vi "Timer tengely.vi"(8 "error in (no error)":errorcluster, 11 "Message Queues in":T1) -> (0 "error out":errorcluster, 3 "Message Queue":refnum<queue>)   [LabVIEW 2014]
uses:
  support/Message Queue/Message Queue.lvlib
  support/Message Queue/Enqueue Message (Single).vi
  Engine/Message.ctl
  Teszt/Command.ctl
  Teszt/Teszt.ctl
  <vilib>/ErrorRing/Error Ring.xnode
  <vilib>/Utility/error.llb/Error Cluster From Error Code.vi
  support/Message Queue/Message Cluster.ctl
  support/Message Queue/All Message Queues.ctl
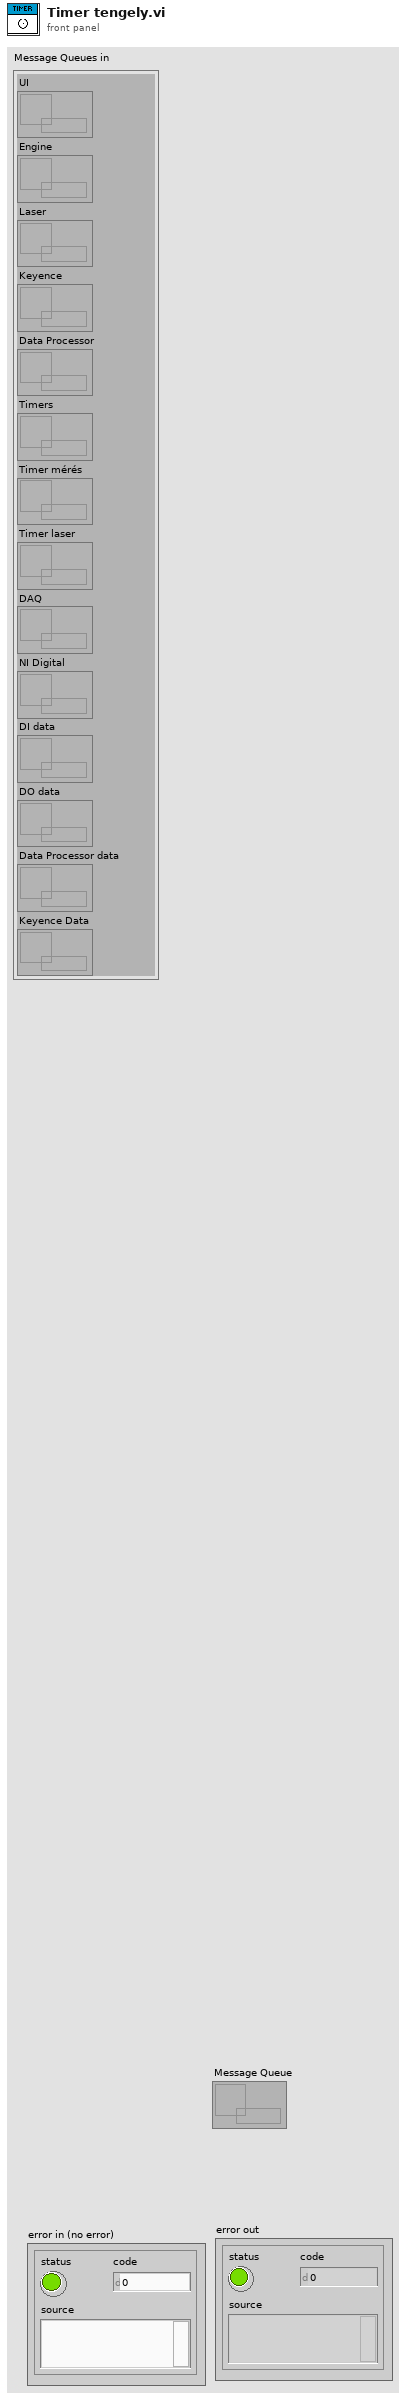
[diagram p1: front panel]
types:
  T1 = typedef "Message Queue.lvlib/All Message Queues.ctl" = cluster{"UI":refnum<queue>, "Engine":refnum<queue>, "Laser":refnum<queue>, "Keyence":refnum<queue>, "Data Processor":refnum<queue>, "Timers":refnum<queue>, "Timer mérés":refnum<queue>, "Timer laser":refnum<queue>, "DAQ":refnum<queue>, "NI Digital":refnum<queue>, "DI data":refnum<queue>, "DO data":refnum<queue>, "Data Processor data":refnum<queue>, "Keyence Data":refnum<queue>}
  T2 = typedef "Teszt.ctl" = cluster{"Thread ID":dbl, "Mérésszám":string, "Mérés/Utasítás":string, "Command":T3, "Min":string, "Max":string, "Aktív?":bool, "Log?":bool, "Kiértékelés":bool, "Etalon 1 exp":bool, "Etalon 2 exp":bool, "Etalon 3 exp":bool, "Etalon 4 exp":bool, "Etalon 5 exp":bool}
  T3 = typedef "Command.ctl" = cluster{"Parancs":string, "Paraméter 1":string, "Paraméter 2":string, "Paraméter 3":string, "Paraméter 4":string, "Paraméter 5":string, "Eredmény":string}
  T4 = typedef "Message.ctl" = cluster{"Thread ID":u16, "Callback":string, "Data":variant, "Error":errorcluster}
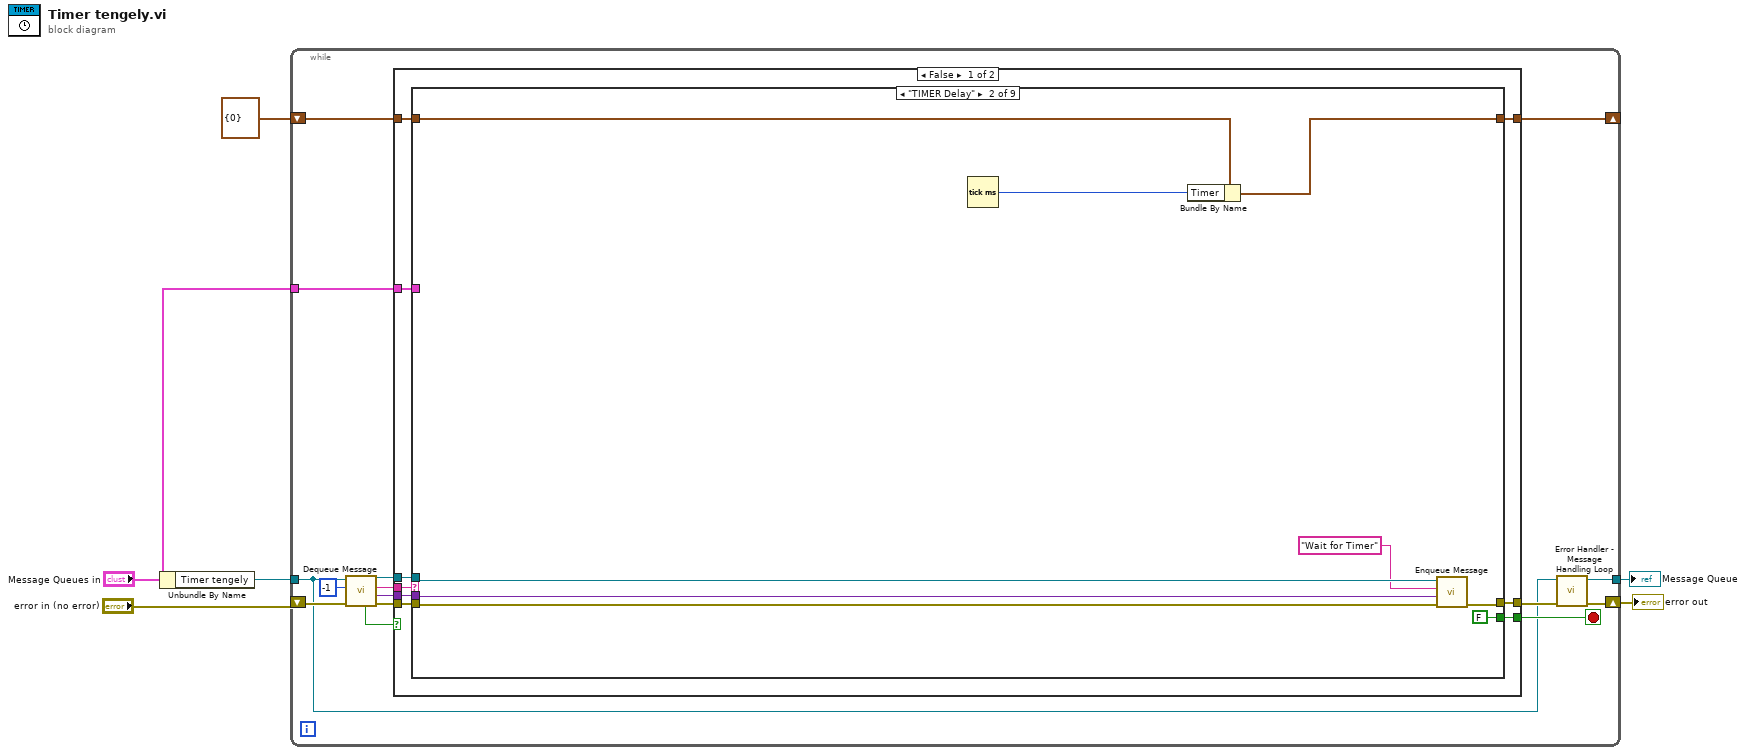
[diagram p0: block diagram]
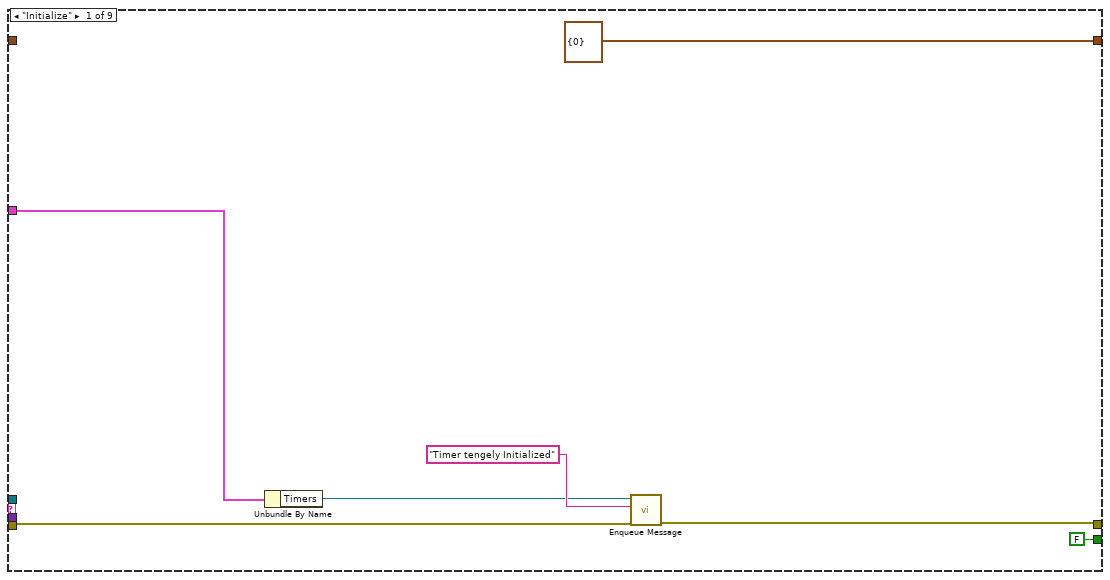
[diagram p2: hidden frame]
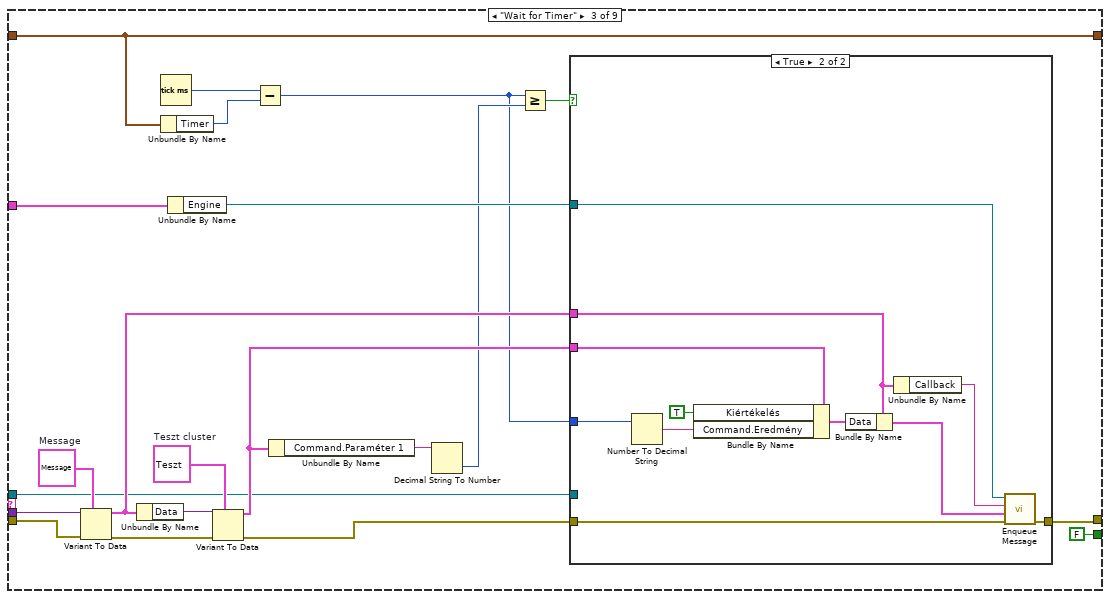
[diagram p3: hidden frame]
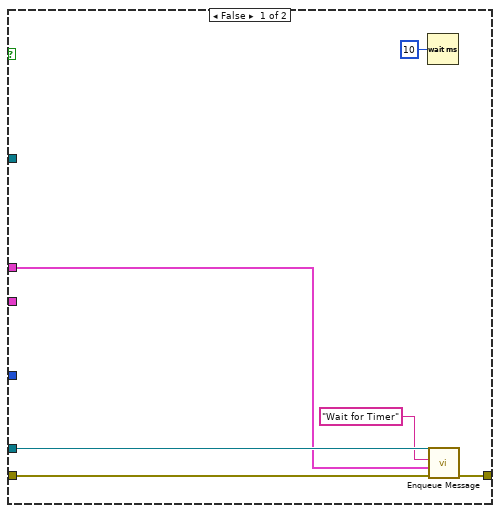
[diagram p4: hidden frame]
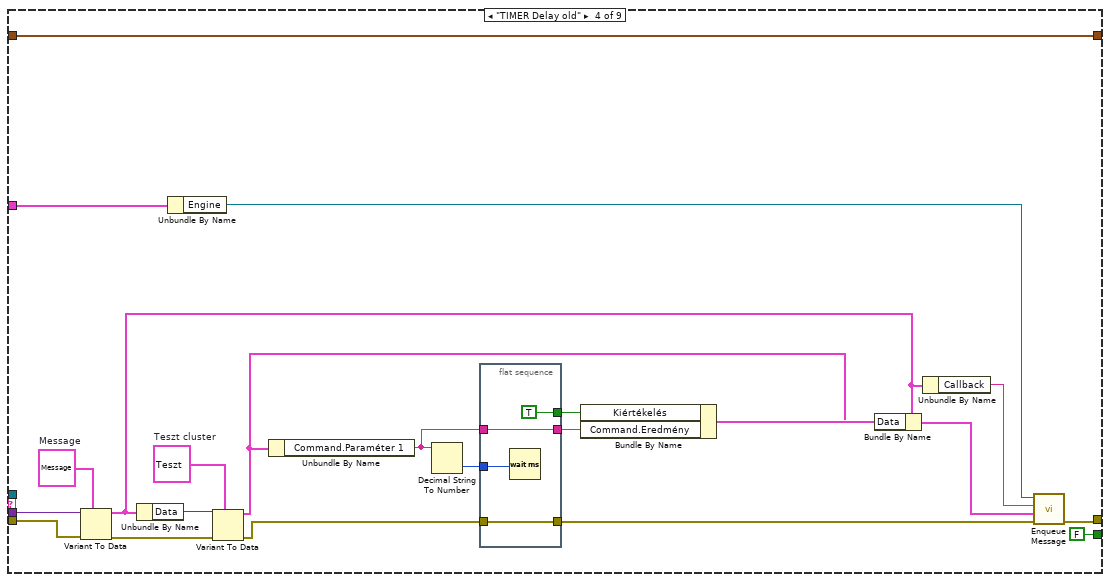
[diagram p5: hidden frame]
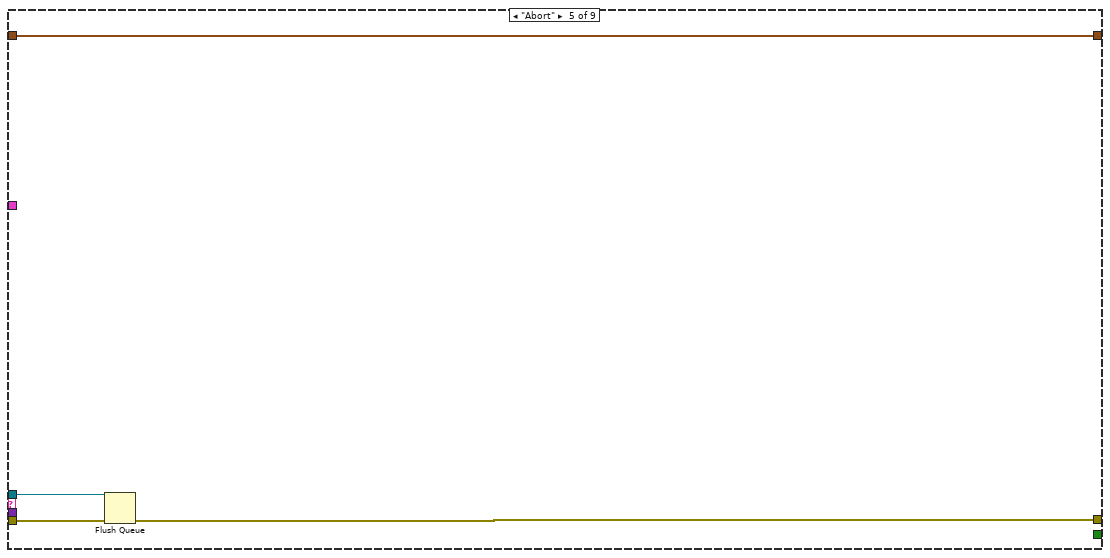
[diagram p6: hidden frame]
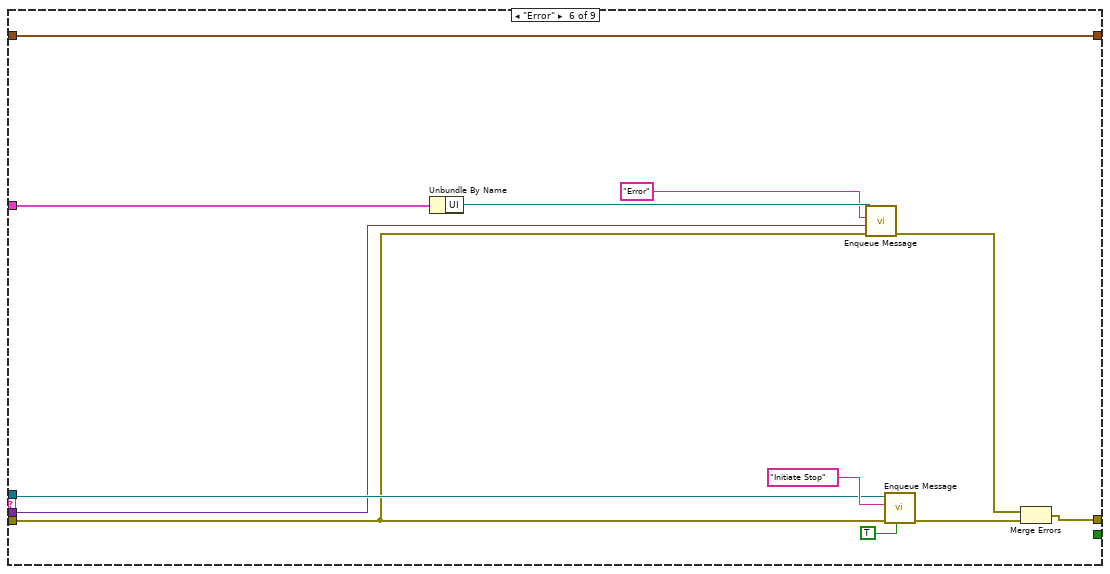
[diagram p7: hidden frame]
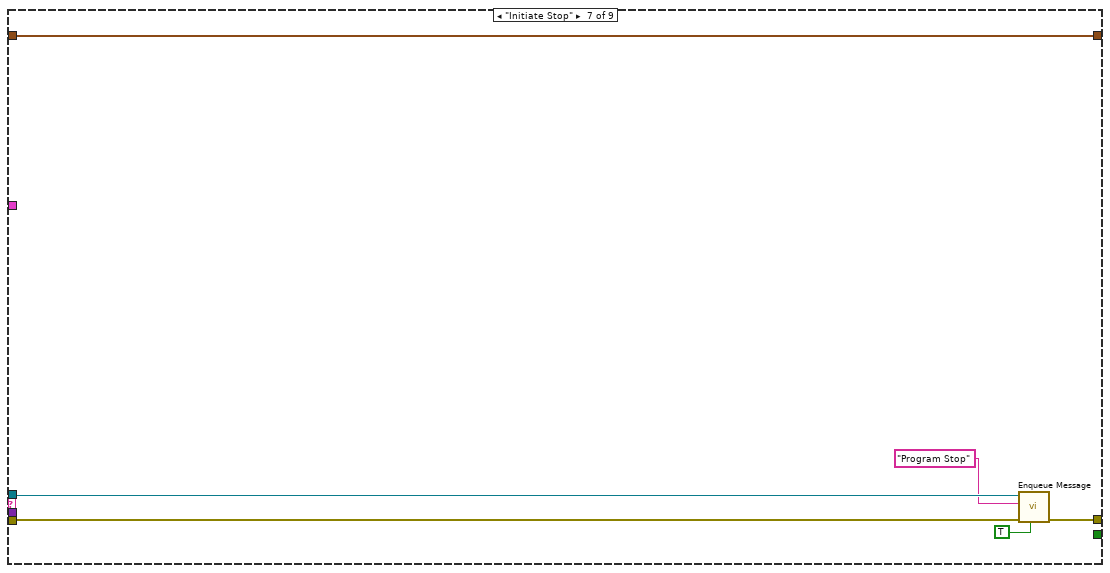
[diagram p8: hidden frame]
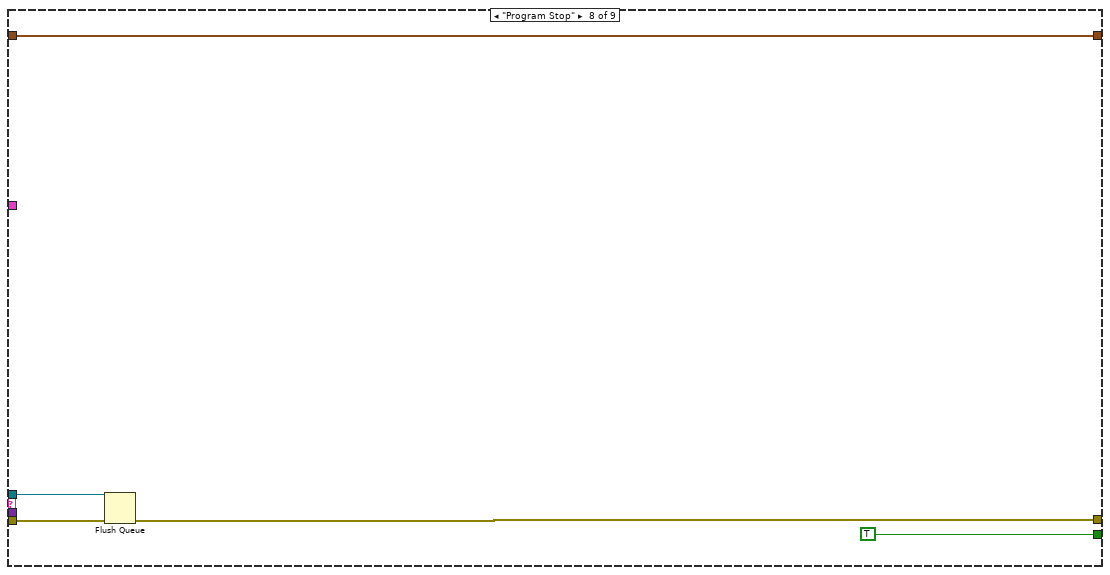
[diagram p9: hidden frame]
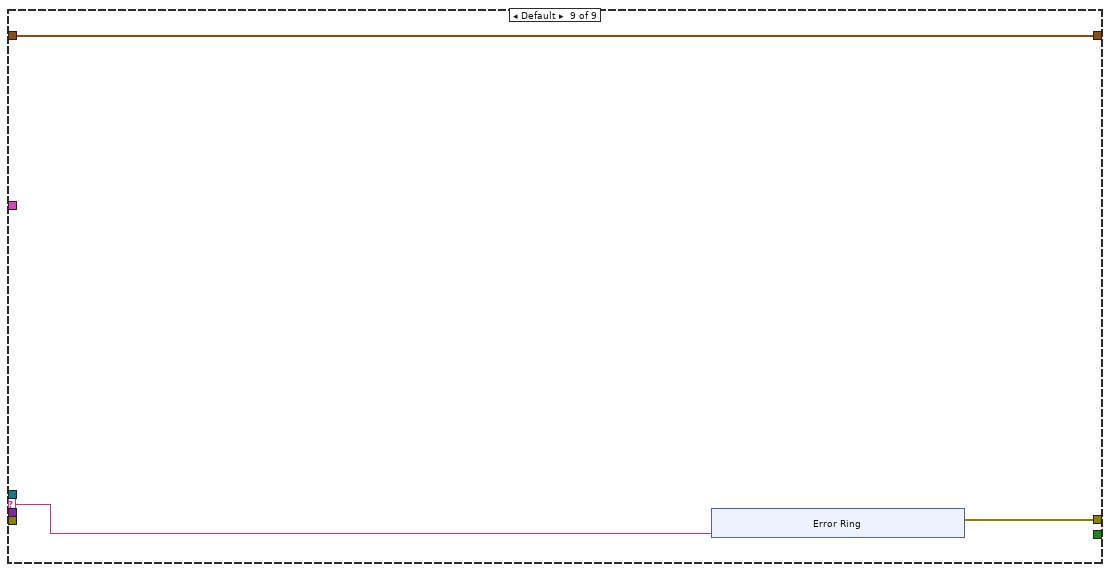
[diagram p10: hidden frame]
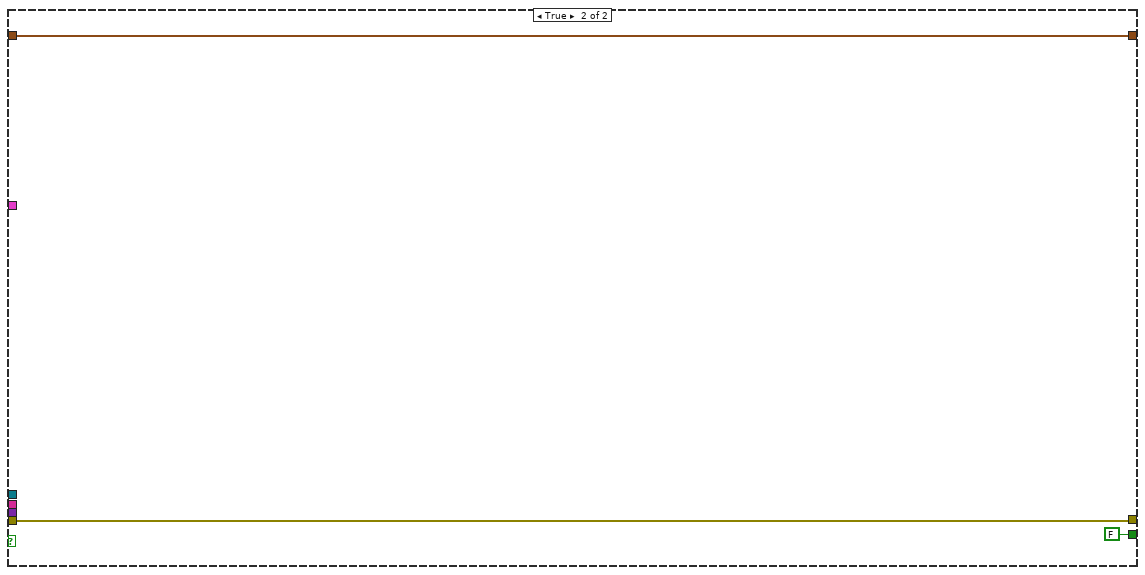
[diagram p11: hidden frame]
diagram:
  n1 = Unbundle By Name("Message Queues in") -> ("Timer tengely"=w3:refnum<queue>)
  n2 = while {
    tunnel: w3 -> [w9]
    shift-right: [w14] -> _
    shift-left: cluster{"Timer":u32} {"Timer"=0} -> [w7]
    shift-right: [w12] -> w6
    shift-left: "error in (no error)" -> [w21]
    tunnel: "Message Queues in" -> [w10]
    tunnel: [w8] -> w2
    stop <- w17 stop-if-true
    n3 = call "Dequeue Message.vi"("error in (no error)"=w21, "timeout in ms (-1)"=-1, "Message Queue"=w9) -> ("error out"=w19:errorcluster, "Message Data"=w13:variant, "Message"=w20:string, "dup Message Queue"=w18:refnum<queue>, "timed out?"=w15:bool)  [unwired: 4 in]
    n4 = case shown="False" w15 {
      tunnel: w20 -> [w30 _]
      tunnel: w19 -> [w29 w149]
      tunnel: w18 -> [w28 _]
      tunnel: [w27 FALSE] -> w17
      tunnel: [w26 w149] -> w11
      tunnel: w7 -> [w24 w150]
      tunnel: [w25 w150] -> w14
      tunnel: w13 -> [w23 _]
      tunnel: w10 -> [w22 _]
      frame False {
        n5 = case shown="\"TIMER Delay\"" w30 {
          selector: w30 -> [_ _ _ _ _ _ _ _ w138]
          tunnel: w29 -> [w33 w42 w67 w106 w114 w116 w130 w137 _]
          tunnel: w28 -> [_ w43 w47 _ w113 w118 w129 w136 _]
          tunnel: [w34 w45 w60 w96 w111 w119 w131 w133 w139] -> w26
          tunnel: [FALSE FALSE FALSE FALSE _ _ _ TRUE _] -> w27
          tunnel: [cluster{"Timer":u32} {"Timer"=0} w38 w54 w105 w112 w126 w132 w134 w140] -> w25
          tunnel: w24 -> [_ w39 w54 w105 w112 w126 w132 w134 w140]
          tunnel: w23 -> [_ w44 w65 w103 _ w115 _ _ _]
          tunnel: w22 -> [w32 _ w57 w92 _ w117 _ _ _]
          frame "Initialize" {
            n6 = Unbundle By Name(w32) -> ("Timers"=w35:refnum<queue>)
            n7 = call-poly "Enqueue Message.vi"("error in (no error)"=w33, "Message"="Timer tengely Initialized", "Message Queue"=w35) -> ("error out"=w34:errorcluster)  [unwired: 7 in, 1 out]
          }
          frame "TIMER Delay" {
            n8 = Tick Count (ms)() -> (millisecond timer value=w40:u32)
            n9 = Bundle By Name(cluster=w39, "Timer"=w40) -> (w38:cluster{"Timer":u32})
            n10 = call-poly "Enqueue Message.vi"("error in (no error)"=w42, "Message Data"=w44, "Message"="Wait for Timer", "Message Queue"=w43) -> ("error out"=w45:errorcluster)  [unwired: 6 in, 1 out]
          }
          frame "Wait for Timer" {
            w61 = T2 {"Thread ID"=0.0, "Mérésszám"="", "Mérés/Utasítás"="", "Command"={"Parancs"="", "Paraméter 1"="", "Paraméter 2"="", "Paraméter 3"="", "Paraméter 4"="", "Paraméter 5"="", "Eredmény"=""}, "Min"="", "Max"="", "Aktív?"=FALSE, "Log?"=FALSE, "Kiértékelés"=FALSE, "Etalon 1 exp"=FALSE, "Etalon 2 exp"=FALSE, "Etalon 3 exp"=FALSE, "Etalon 4 exp"=FALSE, "Etalon 5 exp"=FALSE}  # Teszt cluster
            w64 = T4 {"Thread ID"=0, "Callback"="", "Data"=variant, "Error"={"status"=FALSE, "code"=0, "source"=""}}  # Message
            n11 = Variant To Data(error in=w67, type=w64, Variant=w65) -> (data=w58:T4, error out=w62:errorcluster)
            n12 = Unbundle By Name(w58) -> ("Data"=w63:variant)
            n13 = Tick Count (ms)() -> (millisecond timer value=w53:u32)
            n14 = Unbundle By Name(w54) -> ("Timer"=w52:u32)
            n15 = Unbundle By Name(w57) -> ("Engine"=w56:refnum<queue>)
            n16 = Variant To Data(error in=w62, type=w61, Variant=w63) -> (data=w59:T2, error out=w48:errorcluster)
            n17 = Subtract(x=w53, y=w52) -> (x-y=w50:u32)
            n18 = Unbundle By Name(w59) -> ("Command.Paraméter 1"=w55:string)
            n19 = Decimal String To Number(string=w55) -> (number=w51:i32)  [unwired: 2 in, 1 out]
            n20 = Greater Or Equal?(x=w50, y=w51) -> (x >= y?=w49:bool)
            n21 = case shown="True" w49 {
              tunnel: [w73 w82] -> w60
              tunnel: w59 -> [_ w81]
              tunnel: w58 -> [w69 w80]
              tunnel: w56 -> [_ w78]
              tunnel: w50 -> [_ w74]
              tunnel: w48 -> [w71 w75]
              tunnel: w47 -> [w72 _]
              frame False {
                n22 = Wait (ms)(milliseconds to wait=u32 10) -> ()  [unwired: 1 out]
                n23 = call-poly "Enqueue Message.vi"("error in (no error)"=w71, "Message Data"=w69, "Message"="Wait for Timer", "Message Queue"=w72) -> ("error out"=w73:errorcluster)  [unwired: 6 in, 1 out]
              }
              frame True {
                n24 = Number To Decimal String(number=w74) -> (decimal integer string=w76:string)  [unwired: 1 in]
                n25 = Bundle By Name(cluster=w81, "Kiértékelés"=TRUE, "Command.Eredmény"=w76) -> (w84:T2)
                n26 = Bundle By Name(cluster=w80, "Data"=w84) -> (w83:T4)
                n27 = Unbundle By Name(w80) -> ("Callback"=w79:string)
                n28 = call-poly "Enqueue Message.vi"("error in (no error)"=w75, "Message Data"=w83, "Message"=w79, "Message Queue"=w78) -> ("error out"=w82:errorcluster)  [unwired: 6 in, 1 out]
              }
            }
          }
          frame "TIMER Delay old" {
            w99 = T2 {"Thread ID"=0.0, "Mérésszám"="", "Mérés/Utasítás"="", "Command"={"Parancs"="", "Paraméter 1"="", "Paraméter 2"="", "Paraméter 3"="", "Paraméter 4"="", "Paraméter 5"="", "Eredmény"=""}, "Min"="", "Max"="", "Aktív?"=FALSE, "Log?"=FALSE, "Kiértékelés"=FALSE, "Etalon 1 exp"=FALSE, "Etalon 2 exp"=FALSE, "Etalon 3 exp"=FALSE, "Etalon 4 exp"=FALSE, "Etalon 5 exp"=FALSE}  # Teszt cluster
            w102 = T4 {"Thread ID"=0, "Callback"="", "Data"=variant, "Error"={"status"=FALSE, "code"=0, "source"=""}}  # Message
            n29 = Variant To Data(error in=w106, type=w102, Variant=w103) -> (data=w94:T4, error out=w100:errorcluster)
            n30 = Unbundle By Name(w94) -> ("Data"=w101:variant)
            n31 = Unbundle By Name(w92) -> ("Engine"=w91:refnum<queue>)
            n32 = Variant To Data(error in=w100, type=w99, Variant=w101) -> (data=w95:T2, error out=w89:errorcluster)
            n33 = Unbundle By Name(w95) -> ("Command.Paraméter 1"=w86:string)
            n34 = Decimal String To Number(string=w86) -> (number=w90:i32)  [unwired: 2 in, 1 out]
            n35 = flat-sequence {
              tunnel: w90 -> [w110]
              tunnel: w89 -> [w109]
              tunnel: [w109] -> w88
              tunnel: [TRUE] -> w87
              tunnel: w86 -> [w107]
              tunnel: [w107] -> w85
              frame #0 {
                n36 = Wait (ms)(milliseconds to wait=w110) -> ()  [unwired: 1 out]
              }
            }
            n37 = Bundle By Name(cluster=w95, "Kiértékelés"=w87, "Command.Eredmény"=w85) -> (w98:T2)
            n38 = Bundle By Name(cluster=w94, "Data"=w98) -> (w97:T4)
            n39 = Unbundle By Name(w94) -> ("Callback"=w93:string)
            n40 = call-poly "Enqueue Message.vi"("error in (no error)"=w88, "Message Data"=w97, "Message"=w93, "Message Queue"=w91) -> ("error out"=w96:errorcluster)  [unwired: 6 in, 1 out]
          }
          frame "Abort" {
            n41 = Flush Queue(queue=w113, error in (no error)=w114) -> (error out=w111:errorcluster)  [unwired: 2 out]
          }
          frame "Error" {
            n42 = Unbundle By Name(w117) -> ("UI"=w123:refnum<queue>)
            n43 = call-poly "Enqueue Message.vi"("error in (no error)"=w116, "Message Data"=w115, "Message"="Error", "Message Queue"=w123) -> ("error out"=w125:errorcluster)  [unwired: 6 in, 1 out]
            n44 = call-poly "Enqueue Message.vi"("Priority Message? (F)"=TRUE, "error in (no error)"=w116, "Message"="Initiate Stop", "Message Queue"=w118) -> ("error out"=w124:errorcluster)  [unwired: 6 in, 1 out]
            n45 = Merge Errors(w125, w124) -> (w119:errorcluster)
          }
          frame "Initiate Stop" {
            n46 = call-poly "Enqueue Message.vi"("Priority Message? (F)"=TRUE, "error in (no error)"=w130, "Message"="Program Stop", "Message Queue"=w129) -> ("error out"=w131:errorcluster)  [unwired: 6 in, 1 out]
          }
          frame "Program Stop" {
            n47 = Flush Queue(queue=w136, error in (no error)=w137) -> (error out=w133:errorcluster)  [unwired: 2 out]
          }
          frame Default {
            n48 = xnode "Error Ring"("parameter 0"=w138) -> ("error out"=w139:errorcluster)
          }
        }
      }
      frame True {
      }
    }
    n49 = call "Error Handler - Message Handling Loop.vi"("error in (no error)"=w11, "Message Queue"=w9) -> ("dup error in"=w12:errorcluster, "dup Message Queue"=w8:refnum<queue>)  [unwired: 8 in]
  }
  "error out" <- w6
  "Message Queue" <- w2
